vi "WaitFor(abort).vi"(1 "abort":refnum<queue>, 4 "Wait For Chamber":bool, 5 "Timeout":dbl, 6 "Wait For Position":bool, 7 "Delay":dbl, 8 "Wait For Field":bool, 9 "Wait For Temperature":bool, 10 "error in (no error)":errorcluster, 11 "Instrument Ref In":refnum<k24>) -> (2 "error out":errorcluster, 3 "Instrument Ref Out":refnum<k24>)   [LabVIEW 2019, in "SubVI.lvlib"]
uses:
  SubVI.lvlib
  ppms-6221&2182-7001/QDInstrument_LabView (1)/QDInstrument.dll
  Instance           2 15Saved   WaitFor .vi
  Instance           1 15Saved   WaitFor .vi
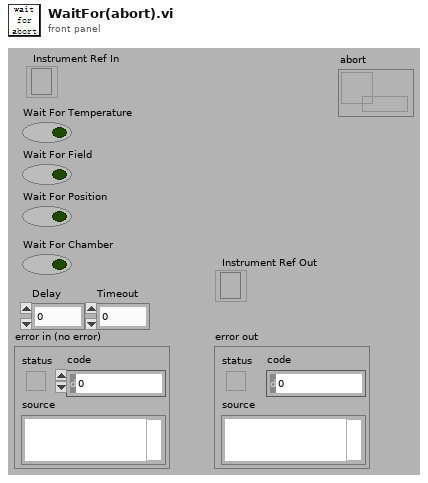
[diagram p1: front panel]
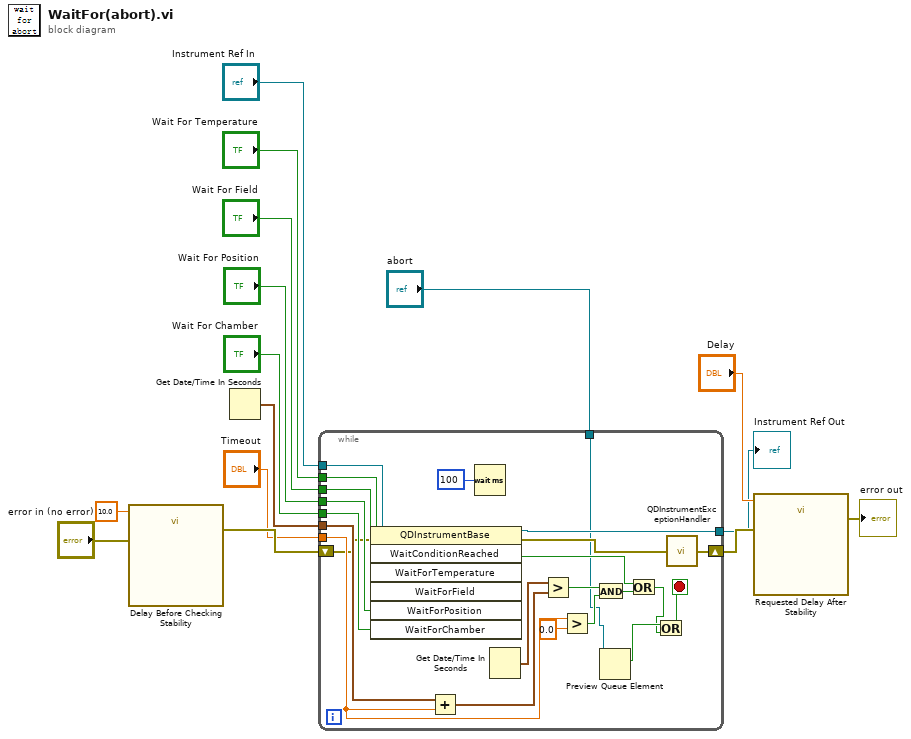
[diagram p0: block diagram]
diagram:
  n1 = call "Delay Before Checking Stability"("error in (no error)"="error in (no error)", "Delay Time (s)"=10.0) -> ("error out"=w6:errorcluster)  [unwired: 9 in]
  n2 = Get Date/Time In Seconds() -> (seconds since 1Jan1904=w5:timestamp)
  n3 = while {
    shift-right: [w20] -> w11
    shift-left: w6 -> [w23]
    tunnel: "Wait For Temperature" -> [w27]
    tunnel: "Wait For Field" -> [w26]
    tunnel: "Wait For Position" -> [w25]
    tunnel: "Wait For Chamber" -> [w24]
    tunnel: w5 -> [w37]
    tunnel: "Timeout" -> [w34]
    tunnel: "Instrument Ref In" -> [w29]
    tunnel: [w28] -> w2
    tunnel: "abort" -> [w19]
    stop <- w16 stop-if-true
    n4 = invoke class="QDInstrumentBase" method="WaitConditionReached"(reference=w29, error in=w23, "WaitForTemperature"=w27, "WaitForField"=w26, "WaitForPosition"=w25, "WaitForChamber"=w24) -> (reference out=w28:refnum<k24>, error out=w21:errorcluster, "WaitConditionReached"=w22:bool)  [unwired: 1 in, 4 out]
    n5 = Add(x=w37, y=w34) -> (x+y=w35:timestamp)
    n6 = Wait (ms)(milliseconds to wait=u32 100) -> ()  [unwired: 1 out]
    n7 = Get Date/Time In Seconds() -> (seconds since 1Jan1904=w36:timestamp)
    n8 = Greater?(x=w36, y=w35) -> (0:w32:bool)
    n9 = Greater?(x=w34, y=0.0) -> (0:w31:bool)
    n10 = And(x=w32, y=w31) -> (x .and. y?=w30:bool)
    n11 = Preview Queue Element(queue=w19) -> (element=w18:bool)  [unwired: 2 in, 3 out]
    n12 = Or(x=w22, y=w30) -> (x .or. y?=w17:bool)
    n13 = Or(x=w18, y=w17) -> (x .or. y?=w16:bool)
    n14 = call "QDInstrumentExceptionHandler.vi"("Error in"=w21) -> ("Error out"=w20:errorcluster)
  }
  "Instrument Ref Out" <- w2
  n15 = call "Requested Delay After Stability"("error in (no error)"=w11, "Delay Time (s)"="Delay") -> ("error out"=→"error out":errorcluster)  [unwired: 9 in]
